vi "TwoEventCases.vi"() -> ()   [LabVIEW 2012]
panel:
  out "布尔":bool
  out "量表":dbl(knob) scale=0.0..10.0
  in  "停止按钮":bool
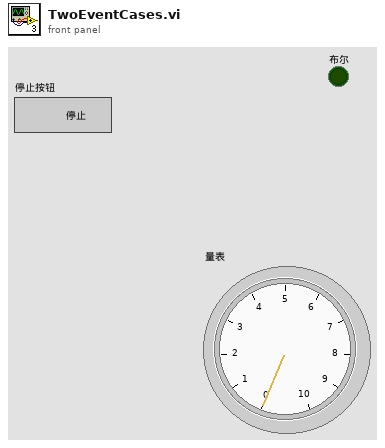
[diagram p1: front panel]
types:
  T1 = typedef "LVPoint32TypeDef.ctl" = cluster{"Horizontal":i32, "Vertical":i32}
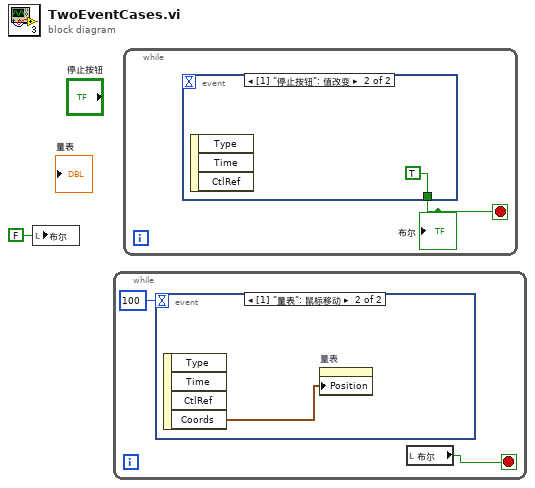
[diagram p0: block diagram]
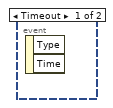
[diagram p2: hidden frame]
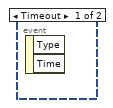
[diagram p3: hidden frame]
diagram:
  n1 = local write "布尔"(FALSE ("布尔")) -> ()
  n2 = while {
    stop <- w3 stop-if-true
    n3 = event shown="[1] \"量表\": 鼠标移动" {
      selector: _ -> [_ _]
      dyn-events: _ -> [_ _]
      timeout: 100 -> [_ _]
      event Timeout {
        n4 = event-data() -> ()  [unwired: 1 in, 2 out]
      }
      event "量表": Mouse Move {
        n5 = event-data() -> ("Coords"=w4:T1)  [unwired: 1 in, 3 out]
        n6 = property on="量表" class="Knob (严格)"("Position"=w4) -> ()  [unwired: 2 in, 2 out]
      }
    }
    n7 = local read "布尔"() -> (w3:bool)
  }
  n8 = while {
    stop <- w5 stop-if-true
    n9 = event shown="[1] \"停止按钮\": 值改变" {
      selector: _ -> [_ _]
      dyn-events: _ -> [_ _]
      timeout: _ -> [_ _]
      tunnel: [_ TRUE] -> w5
      event Timeout {
        n10 = event-data() -> ()  [unwired: 1 in, 2 out]
      }
      event "停止按钮": Value Change {
        n11 = event-data() -> ()  [unwired: 1 in, 3 out]
      }
    }
    "布尔" <- w5
  }
